vi "Get Camera Interface.vi"(8 "error in (no error)":errorcluster, 11 "Dev Ref in":T1 format="%.0x") -> (0 "error out":errorcluster, 2 "Value":string, 3 "Dev Ref out":T1 format="%.0x")   [LabVIEW 2012, in "Image UDP Broadcast Custom Device.lvlib"]
uses:
  Image UDP Broadcast Custom Device.lvlib
  <vilib>/NI Veristand/Custom Device API/Custom Device Item Ref.ctl
  Image UDP Broadcast Global Variable.vi
  <vilib>/NI Veristand/Custom Device API/Get Item Property (String).vi
  <vilib>/NI Veristand/Custom Device API/Custom Device API.lvlib
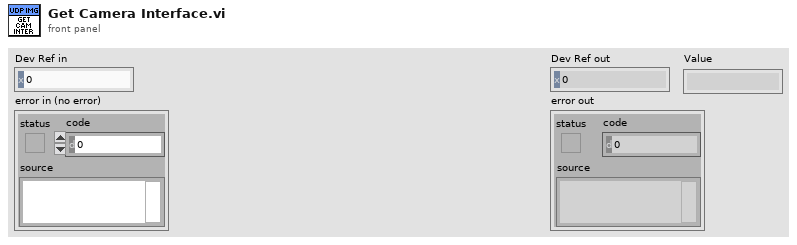
[diagram p1: front panel]
types:
  T1 = typedef "Custom Device API.lvlib/Custom Device Item Ref.ctl" = u64
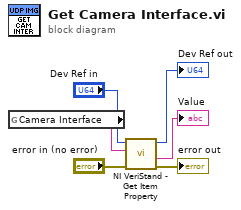
[diagram p0: block diagram]
diagram:
  n1 = global read "Image UDP Broadcast Global Variable.vi" "Camera Interface"() -> (w6:string)
  n2 = call-poly <vilib>:"NI VeriStand - Get Item Property.vi"("error in (no error)"="error in (no error)", "Property Name"=w6, "Item Ref in"="Dev Ref in") -> ("error out"=→"error out":errorcluster, "Value"=→"Value":string, "Item Ref out"=→"Dev Ref out":T1)  [unwired: 5 in, 1 out]
